vi "svc_Create X Array from x0 dx and length.vi"(9 "dx":dbl=1.0, 10 "x0":dbl, 11 "length":i32=1024) -> (3 "X":dbl[](array[numeric]))   [LabVIEW 2017]
doc: "Converts waveform parameters to an explicit X array. Start (t0, x0, f0, etc.), increment (dt, dx, df, etc.), and the number of samples are used to create a ramp of X values that can be used for processing or as the X component when building an XY output data type."
uses:
  <vilib>/Analysis/1siggen.llb/Ramp Pattern by Samples.vi
  <vilib>/Analysis/NI_AALBase.lvlib
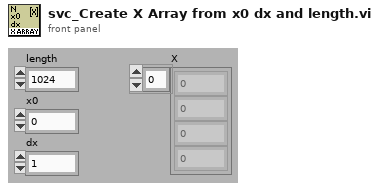
[diagram p1: front panel]
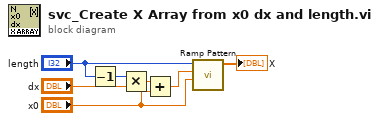
[diagram p0: block diagram]
diagram:
  n1 = Decrement(x="length") -> (x-1=w4:i32)
  n2 = Multiply(x=w4, y="dx") -> (x*y=w2:dbl)
  n3 = Add(x=w2, y="x0") -> (x+y=w1:dbl)
  n4 = call-poly <vilib>:"Ramp Pattern.vi"("start"="x0", "end"=w1, "samples"="length") -> ("Ramp Pattern"=→"X":dbl[])  [unwired: 7 in, 1 out]
